vi "Load Config.vi"(6 "Constants":refnum<class "Sequence Constants.lvclass">, 8 "error in (no error)":refnum<class "MultiErrors.lvclass">, 10 "Config Element":refnum<class "Config Element.lvclass">, 11 "Expression Condition Config in":refnum<class "Expression Condition Config.lvclass">) -> (0 "error out":refnum<class "MultiErrors.lvclass">, 3 "Expression Condition Config out":refnum<class "Expression Condition Config.lvclass">)   [LabVIEW 2020, in "VolatusSeqConfig.lvlib" / "Expression Condition Config.lvclass"]
uses:
  Expression Condition Config.lvclass
  VolatusErrorUtilities/MultiErrors/MultiErrors.lvclass
  lv-cdm/CDM-Config/Config Element/Config Element.lvclass
  Expression Condition Config.lvclass/Expression Condition Config.ctl
  Sequence Constants/Sequence Constants.lvclass
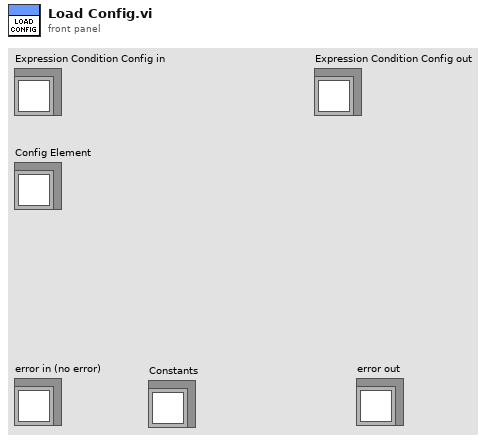
[diagram p1: front panel]
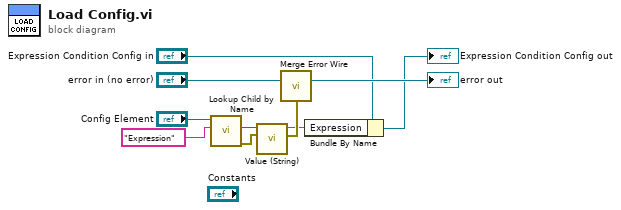
[diagram p0: block diagram]
diagram:
  n1 = call "Lookup Child by Name.vi"("Name"="Expression", "Config Element in"="Config Element") -> ("error out"=w1:errorcluster, "Child"=w4:refnum<class "Config Element.lvclass">)  [unwired: 6 in, 2 out]
  n2 = call "Value (String).vi"("error in (no error)"=w1, "Config Element in"=w4) -> ("error out"=w9:errorcluster, "String Value"=w2:string)  [unwired: 8 in]
  n3 = call "Merge Error Wire.vi"("error in (no error)"=w9, "MultiErrors in"="error in (no error)") -> ("MultiErrors out"=→"error out":refnum<class "MultiErrors.lvclass">)  [unwired: 13 in]
  n4 = Bundle By Name(cluster="Expression Condition Config in", "Expression"=w2) -> (→"Expression Condition Config out":refnum<class "Expression Condition Config.lvclass">)
